vi "MatrixHelper_CoerceSize.vi"(9 "Columns":i32, 10 "Rows":i32, 11 "input matrix":T1) -> (3 "output matrix":T1)   [LabVIEW 2019, in "Trajectory_Library.lvlib"]
doc: "Creates a new LINEAR SYSTEM data cluster with the specified values. \n\n\nInputs: \n - XXX -- XXX.\n\nOutputs:\n - XXX -- XXX."
uses:
  Trajectory_Library.lvlib
  <vilib>/Analysis/Matrix/Datatypes/RealMatrix.ctl
  <vilib>/Analysis/Matrix/NI_Matrix.lvlib
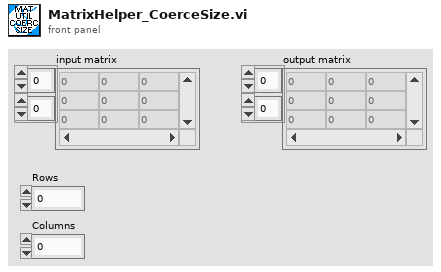
[diagram p1: front panel]
types:
  T1 = typedef "NI_Matrix.lvlib/RealMatrix.ctl" = dbl[][]
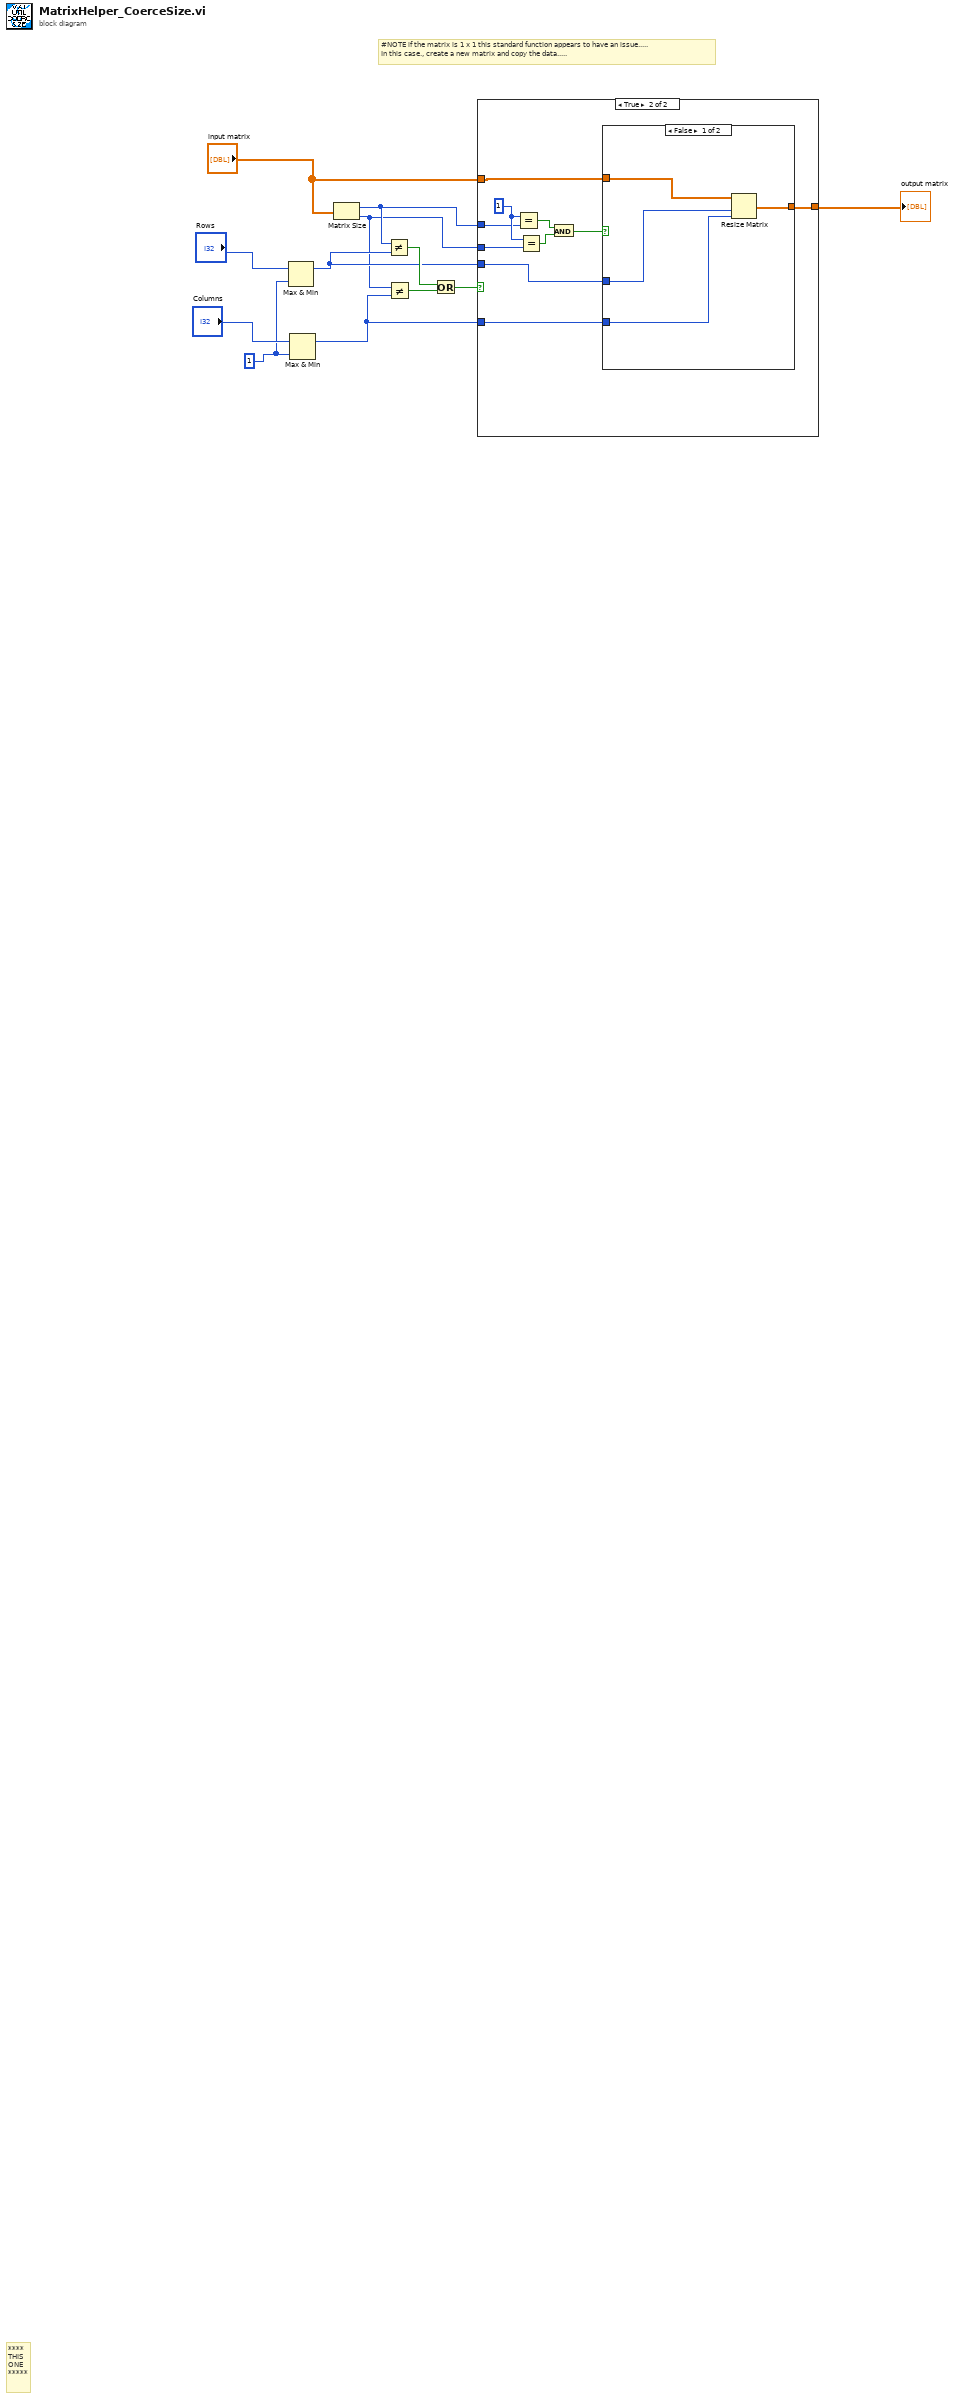
[diagram p0: block diagram]
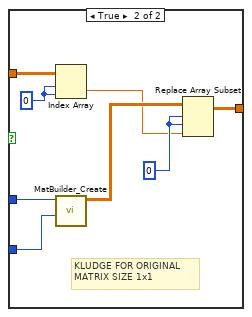
[diagram p3: hidden frame]
diagram:
  w5 = 1 ("y")
  # "#NOTE if the matrix is 1 x 1 this standard function appears to have an issue.....\nIn this case., create a new matrix and copy the data....."
  # "****\nTHIS\nONE\n*****"
  n1 = Max & Min(x="Rows", y=w5) -> (max(x,y)=w4:i32)  [unwired: 1 out]
  n2 = Max & Min(x="Columns", y=w5) -> (max(x,y)=w3:i32)  [unwired: 1 out]
  n3 = Matrix Size(0:"input matrix") -> (1:w2:i32, 2:w1:i32)
  n4 = Not Equal?(x=w2, y=w4) -> (x != y?=w11:bool)
  n5 = Not Equal?(x=w1, y=w3) -> (x != y?=w10:bool)
  n6 = Or(x=w11, y=w10) -> (x .or. y?=w12:bool)
  n7 = case shown="True" w12 {
    tunnel: "input matrix" -> [w13 w15]
    tunnel: [w13 w14] -> w8
    tunnel: w4 -> [_ w17]
    tunnel: w3 -> [_ w16]
    tunnel: w2 -> [_ w22]
    tunnel: w1 -> [_ w21]
    frame False {
    }
    frame True {
      w23 = 1 ("y")
      n8 = Equal?(x=w23, y=w22) -> (x = y?=w19:bool)
      n9 = Equal?(x=w23, y=w21) -> (x = y?=w20:bool)
      n10 = And(x=w19, y=w20) -> (x .and. y?=w18:bool)
      n11 = case shown="False" w18 {
        tunnel: w17 -> [w25 w35]
        tunnel: w16 -> [w24 w34]
        tunnel: w15 -> [w26 w33]
        tunnel: [w27 w30] -> w14
        frame False {
          n12 = Resize Matrix(1:w24, 2:w25, 4:w26) -> (0:w27:T1)
        }
        frame True {
          w29 = 0 ("disabled index (row)")
          w32 = 0 ("index (row)")
          # "KLUDGE FOR ORIGINAL\nMATRIX SIZE 1x1"
          n13 = Index Array(array=w33, index (row)=w32, index (col)=w32) -> (element=w28:dbl)
          n14 = call "MatBuilder_Create.vi"("Columns"=w34, "Rows"=w35) -> ("output matrix"=w31:T1)  [unwired: 9 in]
          n15 = Replace Array Subset(array=w31, new element=w28, index (row)=w29, index (col)=w29) -> (w30:T1)
        }
      }
    }
  }
  "output matrix" <- w8
